vi "Ramsete.vi"(4 "POSE TOL":dbl=0.02, 5 "B":dbl=2.0, 6 "Enabled":bool=TRUE, 7 "ZETA":dbl=0.7, 8 "DesiredAngularVelocity":dbl, 9 "DesiredLinearVelocity":dbl, 10 "DesiredPOSE":T1, 11 "CurrentPOSE":T1) -> (0 "Err Pose":T1, 1 "AtReference":bool, 3 "CHASSIS Speeds":T4)   [LabVIEW 2019, in "PathExecution_Library.lvlib"]
doc: "Ramsete is a nonlinear time-varying feedback controller for unicycle models\n that drives the model to a desired pose along a two-dimensional trajectory.\n Why would we need a nonlinear control law in addition to the linear ones we\n have used so far like PID? If we use the original approach with PID\n controllers for left and right position and velocity states, the controllers\n only deal with the local pose. If the robot deviates from the path, there is\n no way for the controllers to correct and the robot may not reach the desired\n global pose. This is due to multiple endpoints existing for the robot which\n have the same encoder path arc lengths.\n\n Instead of using wheel path arc lengths (which are in the robot's local\n coordinate frame), nonlinear controllers like pure pursuit and Ramsete use\n global pose. The controller uses this extra information to guide a linear\n reference tracker like the PID controllers back in by adjusting the\n references of the PID controllers.\n\n The paper \"Control of Wheeled Mobile Robots: An Experimental Overview\"\n describes a nonlinear controller for a wheeled vehicle with unicycle-like\n kinematics; a global pose consisting of x, y, and theta; and a desired pose\n consisting of x_d, y_d, and theta_d. We call it Ramsete because that's the\n acronym for the title of the book it came from in Italian (\"Robotica\n Articolata e Mobile per i SErvizi e le TEcnologie\").\n\n See <https://file.tavsys.net/control/controls-engineering-in-frc.pdf> section\n on Ramsete unicycle controller for a derivation and analysis.\n\nConcepts for this code were incorportated from the WPILIB ramsete class. \n\n Copyright (c) 2019-2020 FIRST. All Rights Reserved. \n Open Source Software - may be modified and shared by FRC teams. The code \n must be accompanied by the FIRST BSD license file in the root directory of \n the project."
uses:
  PathExecution_Library.lvlib
  POSE.ctl
  TRANSLATION.ctl
  ROTATION.ctl
  CHASSIS.ctl
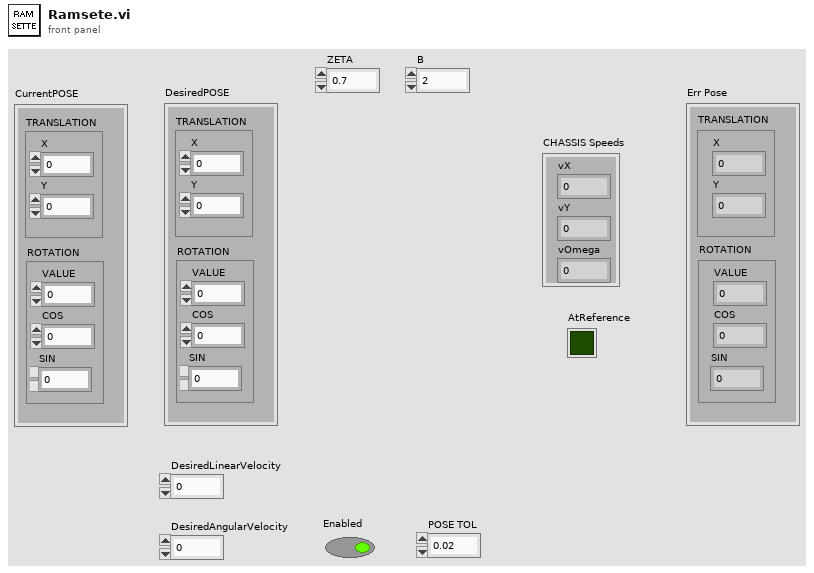
[diagram p1: front panel]
types:
  T1 = typedef "PathExecution_Library.lvlib/POSE.ctl" = cluster{"TRANSLATION":T2, "ROTATION":T3}
  T2 = typedef "PathExecution_Library.lvlib/TRANSLATION.ctl" = cluster{"X":dbl, "Y":dbl}
  T3 = typedef "PathExecution_Library.lvlib/ROTATION.ctl" = cluster{"VALUE":dbl, "COS":dbl, "SIN":dbl}
  T4 = typedef "PathExecution_Library.lvlib/CHASSIS.ctl" = cluster{"vX":dbl, "vY":dbl, "vOmega":dbl}
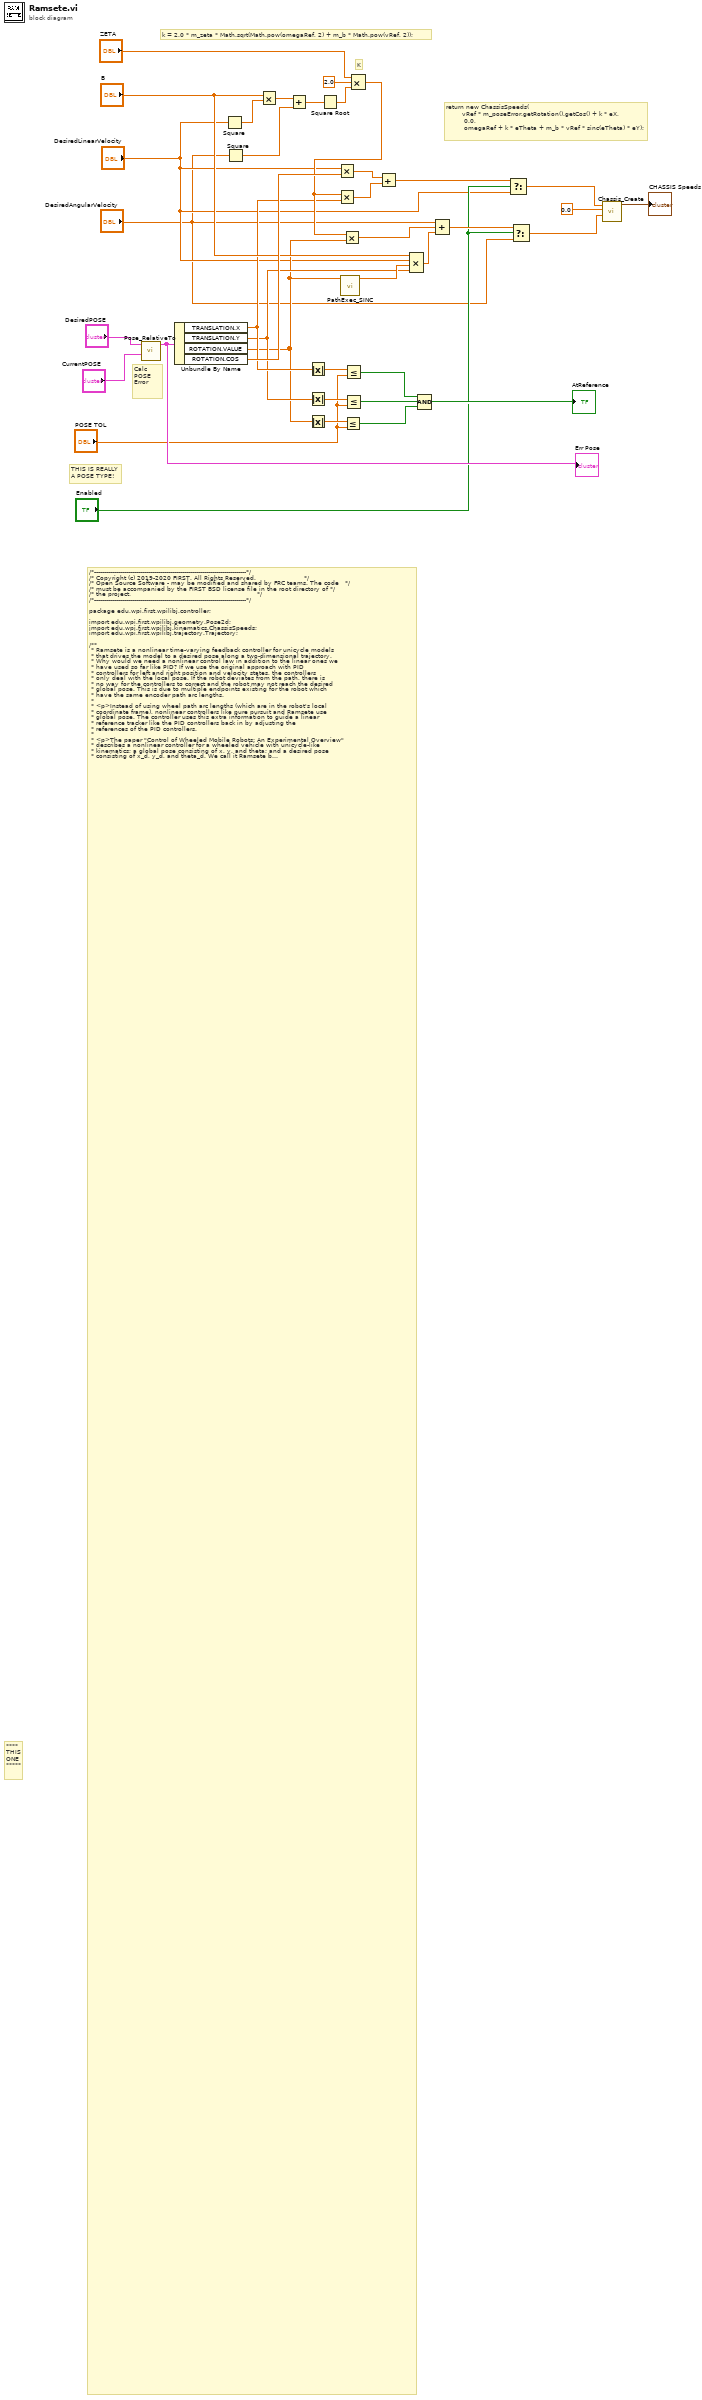
[diagram p0: block diagram]
diagram:
  # "THIS IS REALLY\nA POSE TYPE!"
  # "return new ChassisSpeeds(\n        vRef * m_poseError.getRotation().getCos() + k * eX,\n         0.0,\n         omegaRef + k * eTheta + m_b * vRef * sinc(eTheta) * eY);"
  # "K"
  # "****\nTHIS\nONE\n*****"
  # "k = 2.0 * m_zeta * Math.sqrt(Math.pow(omegaRef, 2) + m_b * Math.pow(vRef, 2));"
  # "Calc POSE\nError"
  # "/*----------------------------------------------------------------------------*/\n/* Copyright (c) 2019-2020 FIRST. All Rights Reserved.                        */\n/* Open Source Software - may be modified and shared by FRC teams. The code   */\n/* must be accompanied by the FIRST BSD license file in the root directory of */\n/* the project.                                                               */\n/*----------------------------------------------------------------------------*/\n\npackage edu.wpi.first.wpilibj.controller;\n\nimport edu.wpi.first.wpilibj.geometry.Pose2d;\nimport edu.wpi.first.wpilibj.kinematics.ChassisSpeeds;\nimport edu.wpi.first.wpilibj.trajectory.Trajectory;\n\n/**\n * Ramsete is a nonlinear time-varying feedback controller for unicycle models\n * that drives the model to a desired pose along a two-dimensional trajectory.\n * Why would we need a nonlinear control law in addition to the linear ones we\n * have used so far like PID? If we use the original approach with PID\n * controllers for left and right position and velocity states, the controllers\n * only deal with the local pose. If the robot deviates from the path, there is\n * no way for the controllers to correct and the robot may not reach the desired\n * global pose. This is due to multiple endpoints existing for the robot which\n * have the same encoder path arc lengths.\n *\n * <p>Instead of using wheel path arc lengths (which are in the robot's local\n * coordinate frame), nonlinear controllers like pure pursuit and Ramsete use\n * global pose. The controller uses this extra information to guide a linear\n * reference tracker like the PID controllers back in by adjusting the\n * references of the PID controllers.\n *\n * <p>The paper \"Control of Wheeled Mobile Robots: An Experimental Overview\"\n * describes a nonlinear controller for a wheeled vehicle with unicycle-like\n * kinematics; a global pose consisting of x, y, and theta; and a desired pose\n * consisting of x_d, y_d, and theta_d. We call it Ramsete because that's the\n * acronym for the title of the book it came from in Italian (\"Robotica\n * Articolata e Mobile per i SErvizi e le TEcnologie\").\n *\n * <p>See\n * <a href=\"https://file.tavsys.net/control/controls-engineering-in-frc.pdf\">\n * Controls Engineering in the FIRST Robotics Competition</a> section on Ramsete\n * unicycle controller for a derivation and analysis.\n */\n\n// ===============================================================\npublic class RamseteController {\n\n//-----------------------------------------------------------------------------------------------------\n//--------Private data\n  @SuppressWarnings(\"MemberName\")\n  private final double m_b;\n  @SuppressWarnings(\"MemberName\")\n  private final double m_zeta;\n\n  private Pose2d m_poseError = new Pose2d();\n  private Pose2d m_poseTolerance = new Pose2d();\n  private boolean m_enabled = true;\n\n//-----------------------------------------------------------------------------------------------------\n//--------Constructor  ( b, zeta )\n  /**\n   * Construct a Ramsete unicycle controller.\n   *\n   * @param b    Tuning parameter (b &gt; 0) for which larger values make convergence more\n   *             aggressive like a proportional term.\n   * @param zeta Tuning parameter (0 &lt; zeta &lt; 1) for which larger values provide more damping\n   *             in response.\n   */\n  @SuppressWarnings(\"ParameterName\")\n  public RamseteController(double b, double zeta) {\n    m_b = b;\n    m_zeta = zeta;\n  }\n\n//-----------------------------------------------------------------------------------------------------\n//--------Constructor  ( )\n  /**\n   * Construct a Ramsete unicycle controller. The default arguments for\n   * b and zeta of 2.0 and 0.7 have been well-tested to produce desireable\n   * results.\n   */\n  public RamseteController() {\n    this(2.0, 0.7);\n  }\n\n//-----------------------------------------------------------------------------------------------------\n//--------atReference\n  /**\n   * Returns true if the pose error is within tolerance of the reference.\n   */\n  public boolean atReference() {\n    final var eTranslate = m_poseError.getTranslation();\n    final var eRotate = m_poseError.getRotation();\n    final var tolTranslate = m_poseTolerance.getTranslation();\n    final var tolRotate = m_poseTolerance.getRotation();\n    return Math.abs(eTranslate.getX()) < tolTranslate.getX()\n           && Math.abs(eTranslate.getY()) < tolTranslate.getY()\n           && Math.abs(eRotate.getRadians()) < tolRotate.getRadians();\n  }\n\n//-----------------------------------------------------------------------------------------------------\n//--------Set POSE Error\n  /**\n   * Sets the pose error which is considered tolerable for use with\n   * atReference().\n   *\n   * @param poseTolerance Pose error which is tolerable.\n   */\n  public void setTolerance(Pose2d poseTolerance) {\n    m_poseTolerance = poseTolerance;\n  }\n\n//-----------------------------------------------------------------------------------------------------\n//--------calculate ( currentPose, refPOSE, linVEL, ang VEL )\n  /**\n   * Returns the next output of the Ramsete controller.\n   *\n   * <p>The reference pose, linear velocity, and angular velocity should come\n   * from a drivetrain trajectory.\n   *\n   * @param currentPose                        The current pose.\n   * @param poseRef                            The desired pose.\n   * @param linearVelocityRefMeters            The desired linear velocity in meters.\n   * @param angularVelocityRefRadiansPerSecond The desired angular velocity in meters.\n   */\n  @SuppressWarnings(\"LocalVariableName\")\n  public ChassisSpeeds calculate(Pose2d currentPose,\n                                 Pose2d poseRef,\n                                 double linearVelocityRefMeters,\n                                 double angularVelocityRefRadiansPerSecond) {\n    if (!m_enabled) {\n      return new ChassisSpeeds(linearVelocityRefMeters, 0.0, angularVelocityRefRadiansPerSecond);\n    }\n\n    m_poseError = poseRef.relativeTo(currentPose);\n\n    // Aliases for equation readability\n    final double eX = m_poseError.getTranslation().getX();\n    final double eY = m_poseError.getTranslation().getY();\n    final double eTheta = m_poseError.getRotation().getRadians();\n\n    final double vRef = linearVelocityRefMeters;\n    final double omegaRef = angularVelocityRefRadiansPerSecond;\n\n    double k = 2.0 * m_zeta * Math.sqrt(Math.pow(omegaRef, 2) + m_b * Math.pow(vRef, 2));\n\n    return new ChassisSpeeds(vRef * m_poseError.getRotation().getCos() + k * eX,\n                             0.0,\n                             omegaRef + k * eTheta + m_b * vRef * sinc(eTheta) * eY);\n  }\n\n//-----------------------------------------------------------------------------------------------------\n//--------calculate ( currentPose, trajectory )\n  /**\n   * Returns the next output of the Ramsete controller.\n   *\n   * <p>The reference pose, linear velocity, and angular velocity should come\n   * from a drivetrain trajectory.\n   *\n   * @param currentPose  The current pose.\n   * @param desiredState The desired pose, linear velocity, and angular velocity\n   *                     from a trajectory.\n   */\n  @SuppressWarnings(\"LocalVariableName\")\n  public ChassisSpeeds calculate(Pose2d currentPose, Trajectory.State desiredState) {\n    return calculate(currentPose, desiredState.poseMeters, desiredState.velocityMetersPerSecond,\n        desiredState.velocityMetersPerSecond * desiredState.curvatureRadPerMeter);\n  }\n\n//-----------------------------------------------------------------------------------------------------\n//--------enabled\n  /**\n   * Enables and disables the controller for troubleshooting purposes.\n   *\n   * @param enabled If the controller is enabled or not.\n   */\n  public void setEnabled(boolean enabled) {\n    m_enabled = enabled;\n  }\n\n//-----------------------------------------------------------------------------------------------------\n//--------sinc\n  /**\n   * Returns sin(x) / x.\n   *\n   * @param x Value of which to take sinc(x).\n   */\n  @SuppressWarnings(\"ParameterName\")\n  private static double sinc(double x) {\n    if (Math.abs(x) < 1e-9) {\n      return 1.0 - 1.0 / 6.0 * x * x;\n    } else {\n      return Math.sin(x) / x;\n    }\n  }\n}"
  n1 = call "Pose_RelativeTo.vi"("other POSE"="CurrentPOSE", "in POSE"="DesiredPOSE") -> ("out POSE"=w38:T1)  [unwired: 9 in]
  "Err Pose" <- w38
  n2 = Unbundle By Name(w38) -> ("TRANSLATION.X"=w22:dbl, "TRANSLATION.Y"=w21:dbl, "ROTATION.VALUE"=w20:dbl, "ROTATION.COS"=w30:dbl)
  n3 = Square(x="DesiredLinearVelocity") -> (x^2=w37:dbl)
  n4 = Square(x="DesiredAngularVelocity") -> (x^2=w35:dbl)
  n5 = Multiply(x="B", y=w37) -> (x*y=w36:dbl)
  n6 = Add(x=w36, y=w35) -> (x+y=w34:dbl)
  n7 = Absolute Value(x=w22) -> (abs(x)=w17:dbl)
  n8 = Absolute Value(x=w21) -> (abs(x)=w18:dbl)
  n9 = Absolute Value(x=w20) -> (abs(x)=w19:dbl)
  n10 = Square Root(x=w34) -> (sqrt(x)=w33:dbl)
  n11 = Multiply(x="DesiredLinearVelocity", y=w30) -> (x*y=w29:dbl)
  n12 = call "PathExec_SINC.vi"("IN VALUE"=w20) -> ("OUT SINC"=w23:dbl)  [unwired: 10 in]
  n13 = Less Or Equal?(x=w19, y="POSE TOL") -> (x <= y?=w13:bool)
  n14 = Less Or Equal?(x=w17, y="POSE TOL") -> (x <= y?=w15:bool)
  n15 = Less Or Equal?(x=w18, y="POSE TOL") -> (x <= y?=w14:bool)
  n16 = Compound Arithmetic op=MULTIPLY("ZETA", 2.0 ("value"), w33) -> (w27:dbl)
  n17 = Multiply(x=w27, y=w22) -> (x*y=w28:dbl)
  n18 = Multiply(x=w27, y=w20) -> (x*y=w26:dbl)
  n19 = Add(x=w29, y=w28) -> (x+y=w11:dbl)
  n20 = Compound Arithmetic op=MULTIPLY("B", "DesiredLinearVelocity", w23, w21) -> (w24:dbl)
  n21 = Compound Arithmetic op=AND(w15, w14, w13) -> (→"AtReference":bool)
  n22 = Compound Arithmetic op=ADD("DesiredAngularVelocity", w26, w24) -> (w10:dbl)
  n23 = Select(t=w11, s="Enabled", f="DesiredLinearVelocity") -> (s? t:f=w4:dbl)
  n24 = Select(t=w10, s="Enabled", f="DesiredAngularVelocity") -> (s? t:f=w3:dbl)
  n25 = call "Chassis_Create.vi"("vAngular"=w3, "vY"=0.0, "vX"=w4) -> ("CHASSIS"=→"CHASSIS Speeds":T4)  [unwired: 8 in]
